vi "Control Panel.vi"(8 "error in (no error)":errorcluster, 11 "Spectrometer iHR320 in":refnum<class "Spectrometer iHR320.lvclass">) -> (0 "error out":errorcluster, 3 "Spectrometer iHR320 out":refnum<class "Spectrometer iHR320.lvclass">)   [LabVIEW 2009, in "Spectrometer iHR320.lvclass"]
doc: "(Dynamic) A user-level application that simulates the physical front panel of the Instrument. Provide the user with buttons to manually control features of the instrument, and provide indicators of its current state."
uses:
  Spectrometer iHR320.lvclass
  Utility Classes/Scannable/Scannable.lvclass
  Spectrometer iHR320.lvclass/Spectrometer iHR320.ctl
panel:
  in  "Copy actual to set":bool
  in  "Populate fields with member data":bool
  out "Grating":u16(ring)=1 items=["1200"=1, "600"=2]
  in  "Set Grating":bool
  in  "stop":bool
  in  "Read to control":bool
  in  "Read":bool
  in  "Go To Wavelength":bool
  in  "Set Slit":bool
  in  "Grating set":u16(ring)=1 items=["1200"=1, "600"=2]
  out "Wavelength":dbl[unit]
  in  "Wavelength Set":dbl[unit]
  out "Exit Slit":dbl[unit]
  in  "Exit Slit Set":dbl[unit]
  out "Entrance Slit":dbl[unit]
  in  "Entrance  set":dbl[unit]
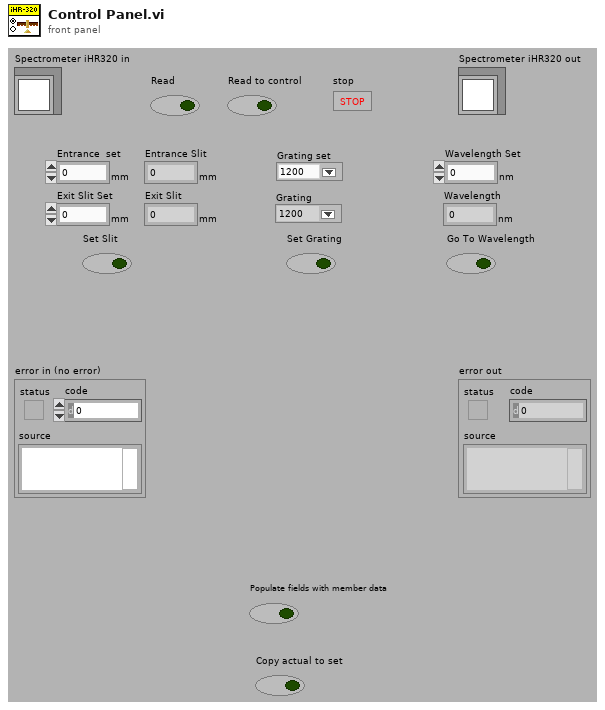
[diagram p1: front panel]
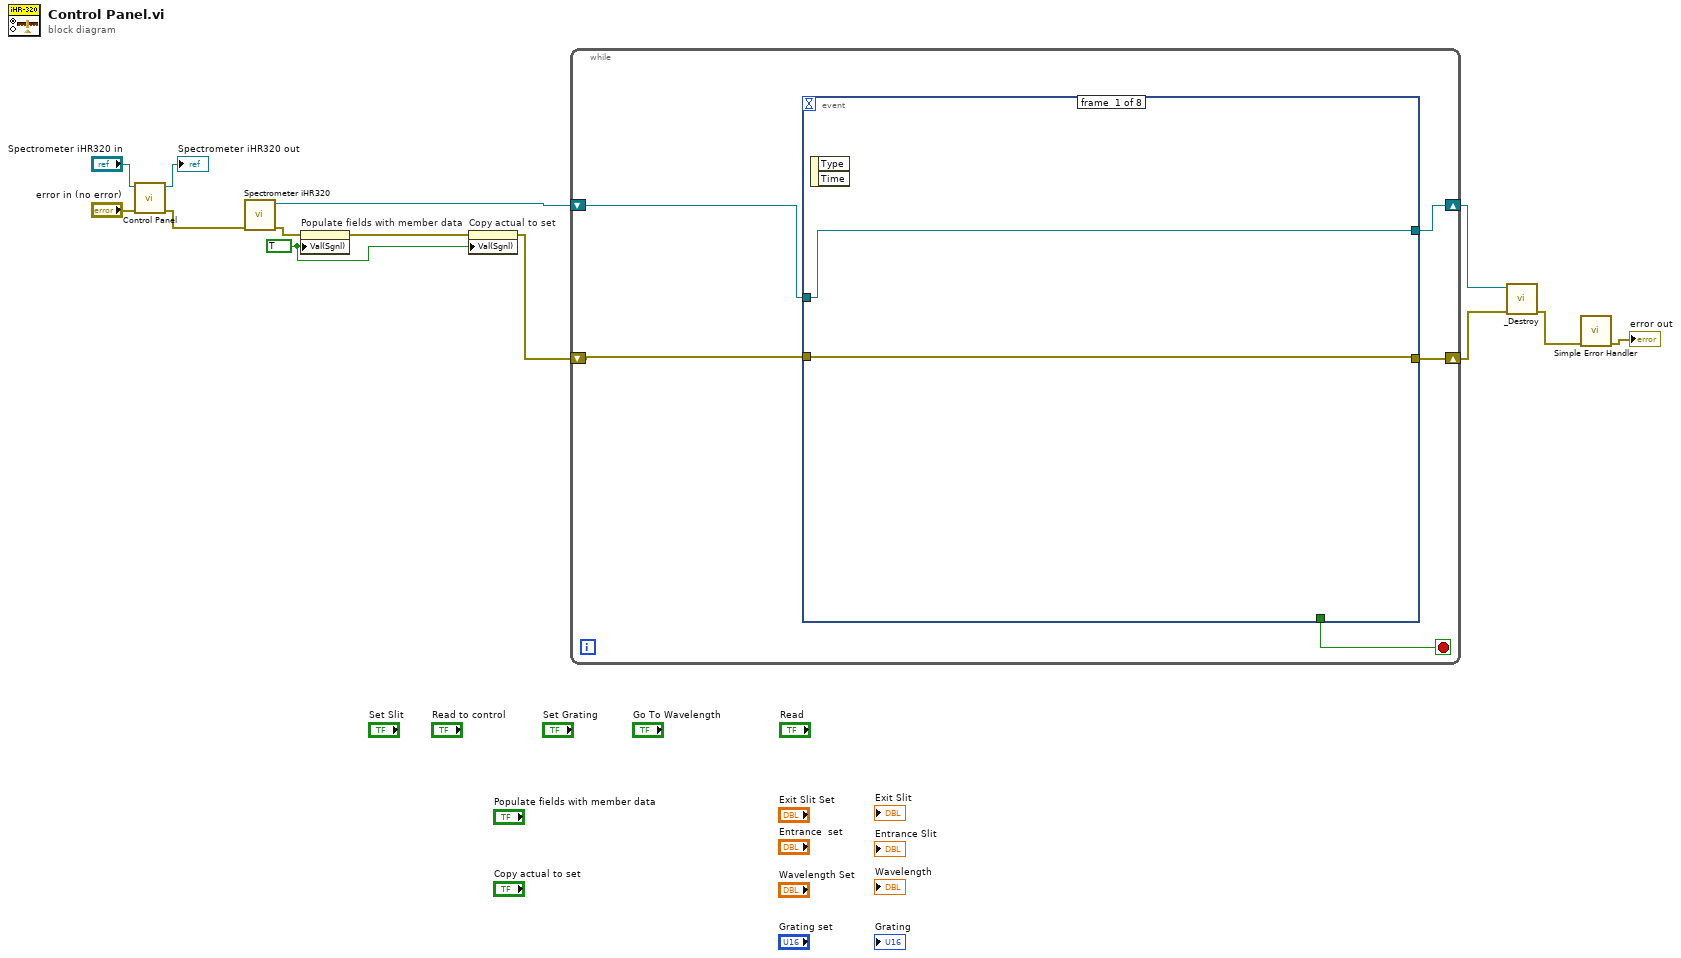
[diagram p0: block diagram]
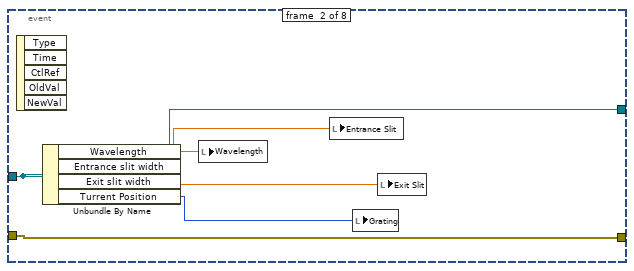
[diagram p2: hidden frame]
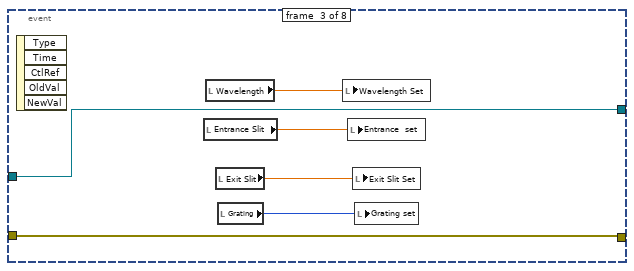
[diagram p3: hidden frame]
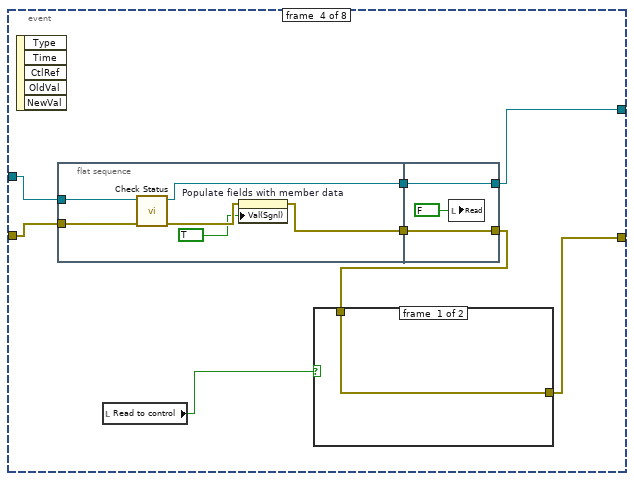
[diagram p4: hidden frame]
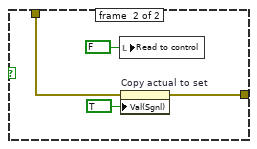
[diagram p5: hidden frame]
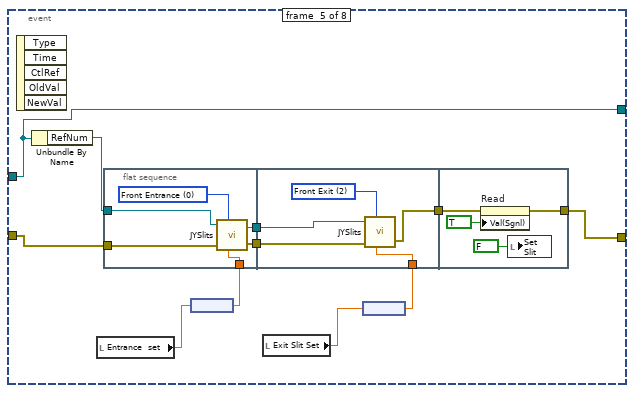
[diagram p6: hidden frame]
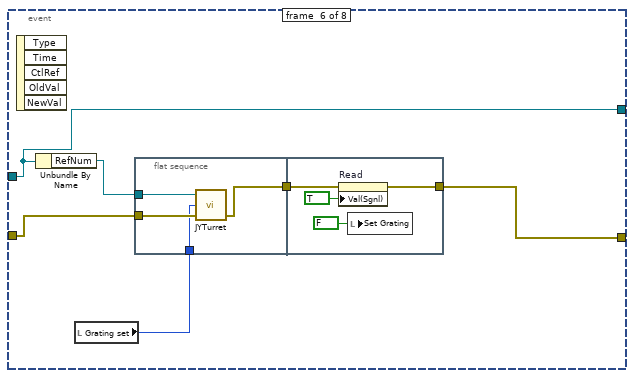
[diagram p7: hidden frame]
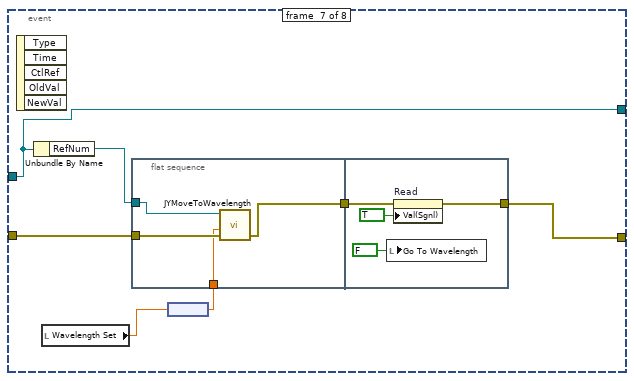
[diagram p8: hidden frame]
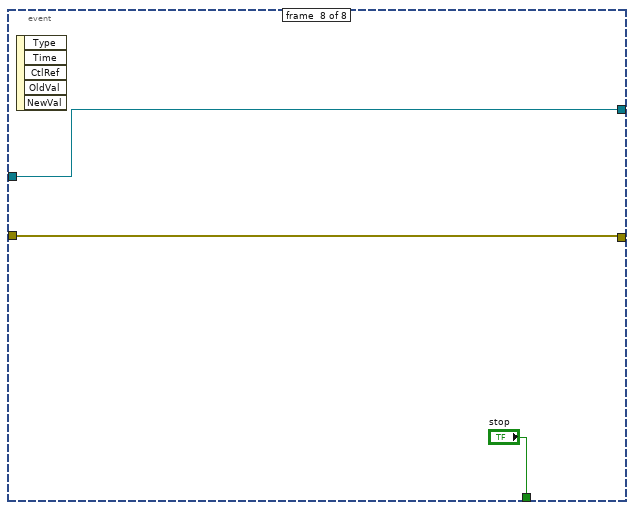
[diagram p9: hidden frame]
diagram:
  w7 = TRUE ("Value (Signaling)")
  n1 = call-parent "Control Panel.vi"("error in (no error)"="error in (no error)", "Instrument in"="Spectrometer iHR320 in") -> ("error out"=w10:errorcluster, "Instrument out"=→"Spectrometer iHR320 out":refnum<class "Spectrometer iHR320.lvclass">)  [unwired: 8 in]
  n2 = call "Spectrometer iHR320.vi"("error in (no error)"=w10) -> ("error out"=w9:errorcluster, "Spectr. iHR320 Out"=w5:refnum<class "Spectrometer iHR320.lvclass">)  [unwired: 9 in]
  n3 = property on="Populate fields with member data" class="Bool (strict)"(error in=w9, "Val(Sgnl)"=w7) -> (error out=w8:errorcluster)  [unwired: 1 in, 1 out]
  n4 = property on="Copy actual to set" class="Bool (strict)"(error in=w8, "Val(Sgnl)"=w7) -> (error out=w6:errorcluster)  [unwired: 1 in, 1 out]
  n5 = while {
    shift-right: [w16] -> w2
    shift-left: w6 -> [w18]
    shift-right: [w15] -> w3
    shift-left: w5 -> [w17]
    stop <- w14 stop-if-true
    n6 = event shown="[3] \"Read\", \"Read to control\": Value Change" {
      selector: _ -> [_ _ _ _ _ _ _ _]
      dyn-events: _ -> [_ _ _ _ _ _ _ _]
      timeout: _ -> [_ _ _ _ _ _ _ _]
      tunnel: w18 -> [w20 w22 w27 w40 w62 w85 w101 w112]
      tunnel: w17 -> [w19 w21 w28 w39 w55 w81 w95 w111]
      tunnel: [w20 w22 w27 w34 w63 w83 w96 w112] -> w16
      tunnel: [w19 w21 w28 w33 w55 w81 w95 w111] -> w15
      tunnel: [_ _ _ _ _ _ _ "stop"] -> w14
      event #0 {
        n7 = event-data() -> ()  [unwired: 1 in, 2 out]
      }
      event #1 {
        n8 = event-data() -> ()  [unwired: 1 in, 5 out]
        n9 = Unbundle By Name(w21) -> ("Wavelength"=w26:dbl[unit], "Entrance slit width"=w25:dbl[unit], "Exit slit width"=w24:dbl[unit], "Turrent Position"=w23:u16)
        n10 = local write "Wavelength"(w26) -> ()
        n11 = local write "Entrance Slit"(w25) -> ()
        n12 = local write "Grating"(w23) -> ()
        n13 = local write "Exit Slit"(w24) -> ()
      }
      event #2 {
        n14 = event-data() -> ()  [unwired: 1 in, 5 out]
        n15 = local read "Entrance Slit"() -> (w31:dbl[unit])
        n16 = local read "Wavelength"() -> (w32:dbl[unit])
        n17 = local read "Exit Slit"() -> (w30:dbl[unit])
        n18 = local read "Grating"() -> (w29:u16)
        n19 = local write "Wavelength Set"(w32) -> ()
        n20 = local write "Entrance  set"(w31) -> ()
        n21 = local write "Exit Slit Set"(w30) -> ()
        n22 = local write "Grating set"(w29) -> ()
      }
      event #3 {
        n23 = event-data() -> ()  [unwired: 1 in, 5 out]
        n24 = flat-sequence {
          tunnel: w40 -> [w51]
          tunnel: w39 -> [w50]
          tunnel: [w47] -> w38
          tunnel: [w46] -> w37
          tunnel: [w53] -> w35
          tunnel: w38 -> [w53]
          tunnel: [w52] -> w33
          tunnel: w37 -> [w52]
          frame #0 {
            n25 = call-dynamic "Check Status.vi"("error in (no error)"=w51, "Spectrometer iHR320 in"=w50) -> ("error out"=w49:errorcluster, "Spectrometer iHR320 out"=w46:refnum<class "Spectrometer iHR320.lvclass">)  [unwired: 6 in, 2 out]
            n26 = property on="Populate fields with member data" class="Bool (strict)"(error in=w49, "Val(Sgnl)"=TRUE ("Value (Signaling)")) -> (error out=w47:errorcluster)  [unwired: 1 in, 1 out]
          }
          frame #1 {
            n27 = local write "Read"(FALSE ("Read")) -> ()
          }
        }
        n28 = local read "Read to control"() -> (w36:bool)
        n29 = case shown="False" w36 {
          tunnel: w35 -> [w41 w43]
          tunnel: [w41 w42] -> w34
          frame #0 {
          }
          frame #1 {
            n30 = local write "Read to control"(FALSE ("Read to control")) -> ()
            n31 = property on="Copy actual to set" class="Bool (strict)"(error in=w43, "Val(Sgnl)"=TRUE ("Value (Signaling)")) -> (error out=w42:errorcluster)  [unwired: 1 in, 1 out]
          }
        }
      }
      event #4 {
        n32 = event-data() -> ()  [unwired: 1 in, 5 out]
        n33 = Unbundle By Name(w55) -> ("RefNum"=w61:refnum<k7>)
        n34 = local read "Entrance  set"() -> (w59:dbl[unit])
        n35 = flat-sequence {
          tunnel: [w70] -> w65
          tunnel: w62 -> [w69]
          tunnel: w61 -> [w68]
          tunnel: [w67] -> w60
          tunnel: w58 -> [w66]
          tunnel: w65 -> [w75]
          tunnel: [w74] -> w64
          tunnel: w60 -> [w73]
          tunnel: w56 -> [w72]
          tunnel: w64 -> [w78]
          tunnel: [w77] -> w63
          frame #0 {
            w71 = u16 0 items=["Front Entrance", "Side Entrance", "Front Exit", "Side Exit", "First Intermediate", "Second Intermediate"] ("Slit")
            n36 = call "JYSlits.vi"("JYMONOLib.IJYMonoReqd In"=w68, "Slit"=w71, "error in (no error)"=w69, "Slit Width"=w66) -> ("JYMONOLib.IJYMonoReqd Out"=w67:refnum<k7>, "error out"=w70:errorcluster)  [unwired: 1 in]
          }
          frame #1 {
            w76 = u16 2 items=["Front Entrance", "Side Entrance", "Front Exit", "Side Exit", "First Intermediate", "Second Intermediate"] ("Slit")
            n37 = call "JYSlits.vi"("JYMONOLib.IJYMonoReqd In"=w73, "Slit"=w76, "error in (no error)"=w75, "Slit Width"=w72) -> ("error out"=w74:errorcluster)  [unwired: 1 in, 1 out]
          }
          frame #2 {
            n38 = property on="Read" class="Bool (strict)"(error in=w78, "Val(Sgnl)"=TRUE ("Value (Signaling)")) -> (error out=w77:errorcluster)  [unwired: 1 in, 1 out]
            n39 = local write "Set Slit"(FALSE ("Set Slit")) -> ()
          }
        }
        n40 = node(w59) -> (w58:dbl)
        n41 = local read "Exit Slit Set"() -> (w57:dbl[unit])
        n42 = node(w57) -> (w56:dbl)
      }
      event #5 {
        n43 = event-data() -> ()  [unwired: 1 in, 5 out]
        n44 = Unbundle By Name(w81) -> ("RefNum"=w86:refnum<k7>)
        n45 = local read "Grating set"() -> (w82:u16)
        n46 = flat-sequence {
          tunnel: w86 -> [w90]
          tunnel: w85 -> [w89]
          tunnel: [w88] -> w84
          tunnel: w82 -> [w87]
          tunnel: w84 -> [w92]
          tunnel: [w91] -> w83
          frame #0 {
            n47 = call "JYTurret.vi"("error in (no error)"=w89, "Grating Index"=w87, "JYMONOLib.IJYMonoReqd In"=w90) -> ("error out"=w88:errorcluster)  [unwired: 2 out]
          }
          frame #1 {
            n48 = property on="Read" class="Bool (strict)"(error in=w92, "Val(Sgnl)"=TRUE ("Value (Signaling)")) -> (error out=w91:errorcluster)  [unwired: 1 in, 1 out]
            n49 = local write "Set Grating"(FALSE ("Set Grating")) -> ()
          }
        }
      }
      event #6 {
        n50 = event-data() -> ()  [unwired: 1 in, 5 out]
        n51 = Unbundle By Name(w95) -> ("RefNum"=w99:refnum<k7>)
        n52 = local read "Wavelength Set"() -> (w98:dbl[unit])
        n53 = flat-sequence {
          tunnel: w101 -> [w105]
          tunnel: [w104] -> w100
          tunnel: w99 -> [w103]
          tunnel: w97 -> [w102]
          tunnel: w100 -> [w107]
          tunnel: [w106] -> w96
          frame #0 {
            n54 = call "JYMoveToWavelength.vi"("error in (no error)"=w105, "Target WL"=w102, "RefNum In"=w103) -> ("error out"=w104:errorcluster)  [unwired: 1 in, 2 out]
          }
          frame #1 {
            n55 = local write "Go To Wavelength"(FALSE ("Go To Wavelength")) -> ()
            n56 = property on="Read" class="Bool (strict)"(error in=w107, "Val(Sgnl)"=TRUE ("Value (Signaling)")) -> (error out=w106:errorcluster)  [unwired: 1 in, 1 out]
          }
        }
        n57 = node(w98) -> (w97:dbl)
      }
      event #7 {
        n58 = event-data() -> ()  [unwired: 1 in, 5 out]
      }
    }
  }
  n59 = call-dynamic "_Destroy.vi"("error in (no error)"=w2, "Spectrometer iHR320 in"=w3) -> ("error out"=w1:errorcluster)  [unwired: 9 in]
  n60 = call <vilib>:"Simple Error Handler.vi"("error in (no error)"=w1) -> ("error out"=→"error out":errorcluster)  [unwired: 4 in, 4 out]
